vi "OPC_UA_Server.vi"() -> (0 "error out":errorcluster, 2 "item node ID":T1, 3 "Refnum out":T2, 4 "item node ID 2":T1, 5 "server endpoint URL":string, 7 "UA Server Running":bool)   [LabVIEW 2025]
uses:
  <vilib>/OPCUA/NI OPC UA Server.lvlib
  <vilib>/OPCUA/server/Create2.vi
  <vilib>/OPCUA/controls/Data Type.ctl
  <vilib>/OPCUA/controls/NodeId.ctl
  <vilib>/OPCUA/controls/OPC UA Server Refnum.ctl
panel:
  out "item node ID 3":T1
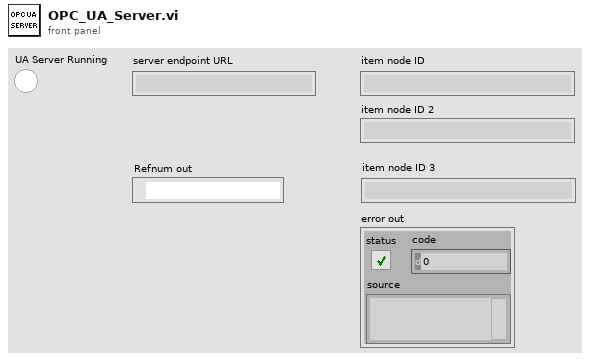
[diagram p1: front panel]
types:
  T1 = typedef "NodeId.ctl" = string
  T2 = typedef "OPC UA Server Refnum.ctl" = refnum<k21>
  T3 = typedef "Data Type.ctl" = u16
  T4 = cluster{"name":string, "data type":T3, "access level":u16, "description":string}
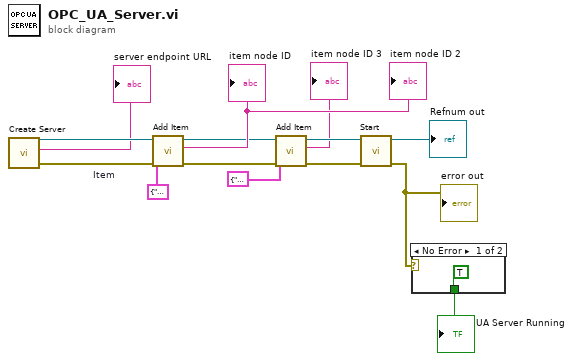
[diagram p0: block diagram]
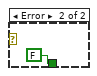
[diagram p2: hidden frame]
diagram:
  w10 = T4 {"name"="Tempreature", "data type"=11, "access level"=3, "description"="TC-01 Data"}  # Item
  n1 = call-poly <vilib>:"Create Server.vi"() -> ("error out"=w9:errorcluster, "server endpoint URL"=→"server endpoint URL":string, "OPC UA server refnum out"=w8:T2)  [unwired: 9 in]
  n2 = call <vilib>:"Add Item.vi"("error in (no error)"=w9, "item"=w10, "OPC UA server refnum in"=w8) -> ("error out"=w5:errorcluster, "item node ID"=→"item node ID" →"item node ID 2":T1, "OPC UA server refnum out"=w4:T2)  [unwired: 4 in, 1 out]
  n3 = call <vilib>:"Add Item.vi"("error in (no error)"=w5, "item"=T4 {"name"="Setpoint Temperature", "data type"=11, "access level"=3, "description"="TC-01 Data Converted"}, "OPC UA server refnum in"=w4) -> ("error out"=w6:errorcluster, "item node ID"=→"item node ID 3":T1, "OPC UA server refnum out"=w3:T2)  [unwired: 4 in, 1 out]
  n4 = call <vilib>:"Start.vi"("error in (no error)"=w6, "OPC UA server refnum in"=w3) -> ("error out"=w13:errorcluster, "OPC UA server refnum out"=→"Refnum out":T2)  [unwired: 7 in, 1 out]
  "error out" <- w13
  n5 = case shown="No Error" w13 {
    tunnel: [TRUE ("Server Status") FALSE ("Server Status")] -> w14
    frame No Error {
    }
    frame Error {
    }
  }
  "UA Server Running" <- w14
